vi "GetDVR.vi"(8 "error in":errorcluster, 11 "BooleanMeasure":refnum<class "BooleanMeasure.lvclass">) -> (0 "error out":errorcluster, 3 "DVRReference":refnum<data-value>)   [LabVIEW 2021, in "ProligentXMLGenerator.lvlib" / "BooleanMeasure.lvclass"]
uses:
  BooleanMeasure.lvclass
  BooleanMeasure.lvclass/BooleanMeasure.ctl
  Data.ctl
  Base/Boolean/Boolean.lvclass
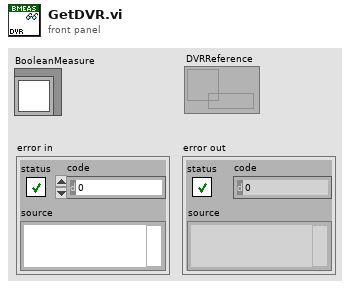
[diagram p1: front panel]
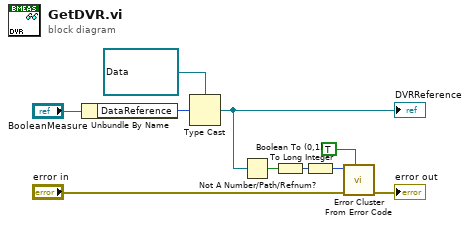
[diagram p0: block diagram]
diagram:
  n1 = Unbundle By Name("BooleanMeasure") -> ("DataReference"=w10:u64)
  n2 = Type Cast(type=refnum<data-value> refnum ("data value reference"), x=w10) -> (*(type *) &x=w6:refnum<data-value>)
  "DVRReference" <- w6
  n3 = Not A Number/Path/Refnum?(number/path/refnum=w6) -> (NaN/Path/Refnum?=w3:bool)
  n4 = Boolean To (0,1)(Boolean=w3) -> (0, 1=w4:i16)
  n5 = To Long Integer(number=w4) -> (32bit integer=w2:i32)
  n6 = call <vilib>:"Error Cluster From Error Code.vi"("show call chain? (False)"=TRUE, "error in (no error)"="error in", "error code (0)"=w2) -> ("error out"=→"error out":errorcluster)  [unwired: 6 in]
